vi "Dir Watch Callback.vi"(4 "User Parameter":T1, 5 "Event Data":cluster{"sender":refnum<k24>, "e":refnum<k24>}, 6 "Control Ref":refnum<k24>, 7 "Event Common Data":T2) -> ()   [LabVIEW 2019]
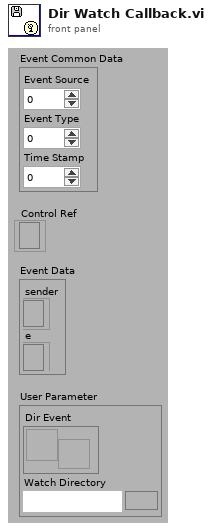
[diagram p1: front panel]
types:
  T1 = cluster{"Dir Event":refnum<user-event>, "Watch Directory":path}
  T2 = cluster{"Event Source":i32, "Event Type":u32, "Time Stamp":u32}
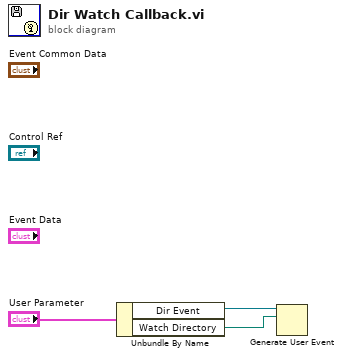
[diagram p0: block diagram]
diagram:
  n1 = Unbundle By Name("User Parameter") -> ("Dir Event"=w2:refnum<user-event>, "Watch Directory"=w1:path)
  n2 = Generate User Event(user event=w2, event data cluster=w1) -> ()  [unwired: 2 in, 2 out]
